vi "Trigger User Event.vi"(7 "priority (normal)":T1, 8 "error in (no error)":errorcluster, 9 "Message Data":variant, 10 "Message":string, 11 "user event in":refnum<user-event>) -> (0 "error out":errorcluster, 3 "user event out":refnum<user-event>)   [LabVIEW 2019]
uses:
  <vilib>/event_ctls.llb/usereventprio.ctl
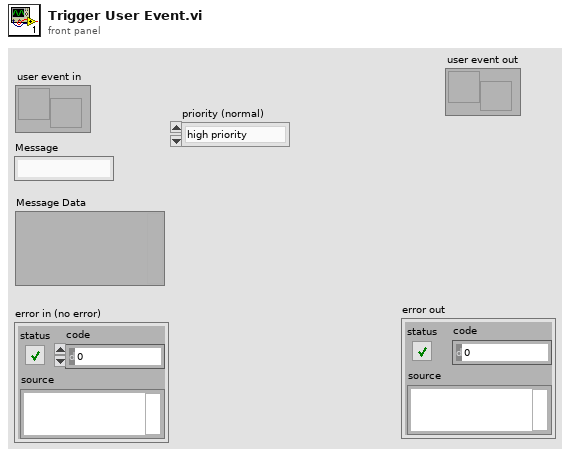
[diagram p1: front panel]
types:
  T1 = typedef "usereventprio.ctl" = enum32{"high priority", "normal priority"}
  T2 = cluster{"Message":string, "Message Data":variant}
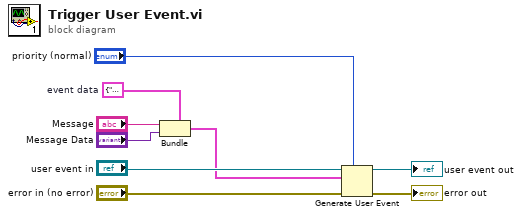
[diagram p0: block diagram]
diagram:
  w2 = T2 {"Message"="", "Message Data"=variant}  # event data
  n1 = Bundle(cluster=w2, "Message"="Message", "Message Data"="Message Data") -> (w1:T2)
  n2 = Generate User Event(priority (normal)="priority (normal)", user event="user event in", event data cluster=w1, error in="error in (no error)") -> (user event out=→"user event out":refnum<user-event>, error out=→"error out":errorcluster)
